vi "niScope Configure Chan Characteristics.vi"(0 "instrument handle":refnum<k15>, 5 "channels":string="0", 7 "input impedance":u32(ring) items=["1 mega ohm"=0, "50 ohms"=2], 9 "maximum input frequency":dbl caption="max input frequency" format="%.2f", 11 "error in":errorcluster) -> (4 "instrument handle out":refnum<k15>, 15 "error out":errorcluster)   [LabVIEW 2013]
doc: "Configures the properties that control the electrical characteristics of the channel. These properties are the input impedance and the bandwidth."
uses:
  niScope_32.dll
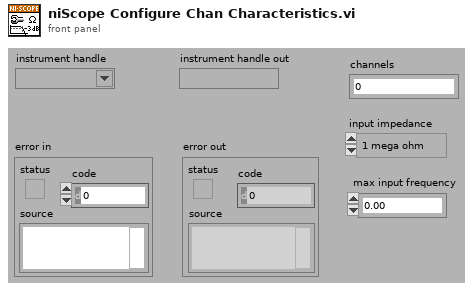
[diagram p1: front panel]
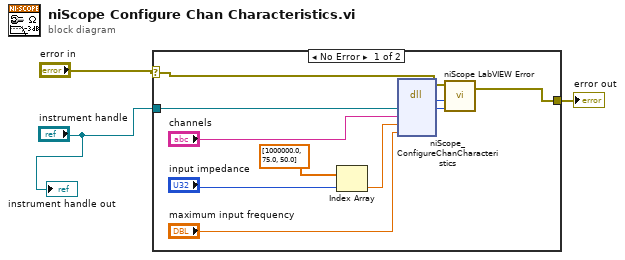
[diagram p0: block diagram]
diagram:
  n1 = case shown="No Error" "error in" {
    selector: "error in" -> [w4 w14]
    tunnel: [w5 w14] -> w2
    tunnel: "instrument handle" -> [w11 _]
    frame No Error {
      n2 = Index Array(array=dbl[] [1000000.0, 75.0, 50.0] ("input impedance arr"), index="input impedance") -> (element=w9:dbl)
      n3 = dll-call lib="niScope_*.*" fn="niScope_ConfigureChanCharacteristics"("instrument handle"=w11, "channel"="channels", "inputImpedance"=w9, "maxInputFrequency"="maximum input frequency") -> ("status"=w7:i32, "instrument handle"=w6:u32)  [unwired: 6 in, 2 out]
      n4 = call <instrlib>:"niScope LabVIEW Error.vi"("instrument handle"=w6, "niScope error code (0)"=w7, "error in (no error)"=w4) -> ("error out"=w5:errorcluster)  [unwired: 2 in]
    }
    frame Error {
    }
  }
  "error out" <- w2
  "instrument handle out" <- "instrument handle"
